vi "K6514_InitializeCharge.vi"(8 "error in (no error)":errorcluster, 11 "VISA resource name":refnum<visa-resource-name>) -> (0 "error out":errorcluster, 3 "VISA resource name out":refnum<visa-resource-name>)   [LabVIEW 2024]
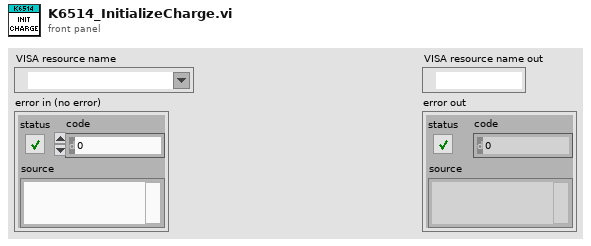
[diagram p1: front panel]
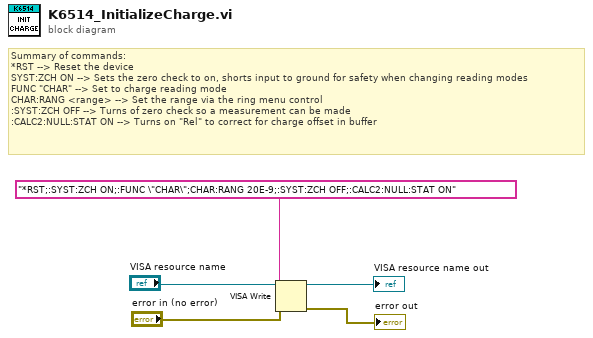
[diagram p0: block diagram]
diagram:
  # "Summary of commands:\n*RST --> Reset the device\nSYST:ZCH ON --> Sets the zero check to on, shorts input to ground for safety when changing reading modes\nFUNC \"CHAR\" --> Set to charge reading mode \nCHAR:RANG <range> --> Set the range via the ring menu control \n:SYST:ZCH OFF --> Turns of zero check so a measurement can be made\n:CALC2:NULL:STAT ON --> Turns on \"Rel\" to correct for charge offset in buffer"
  n1 = VISA Write(VISA resource name="VISA resource name", write buffer="*RST;:SYST:ZCH ON;:FUNC \"CHAR\";CHAR:RANG 20E-9;:SYST:ZCH OFF;:CALC2:NULL:STAT ON", error in (no error)="error in (no error)") -> (VISA resource name out=→"VISA resource name out":refnum<visa-resource-name>, error out=→"error out":errorcluster)  [unwired: 1 out]
